vi "PWM Set Frequency.vi"(7 "pPrecision":u16, 8 "error in (no error)":errorcluster, 9 "pPrescaler":u16, 10 "ChannelMask":u8, 11 "DevHandle":i32) -> (0 "error out":errorcluster, 1 "pPrescaler out":u16, 3 "function return":i32, 5 "pPrecision out":u16)   [LabVIEW 2010, in "usb2pwm.lvlib"]
doc: "int WINAPI PWM_SetFrequency(int DevHandle,unsigned char ChannelMask,unsigned short *pPrescaler,unsigned short *pPrecision);"
uses:
  usb2pwm.lvlib
  libs/msvc_x86/USB2XXX.dll
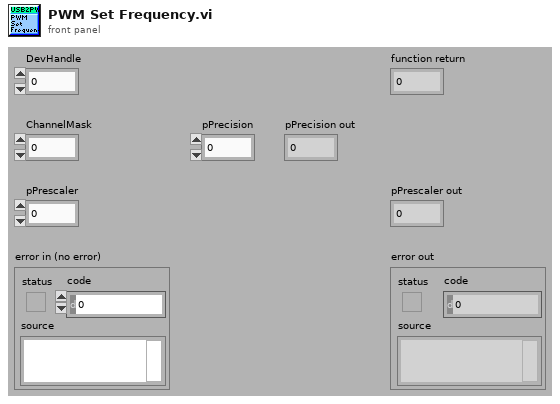
[diagram p1: front panel]
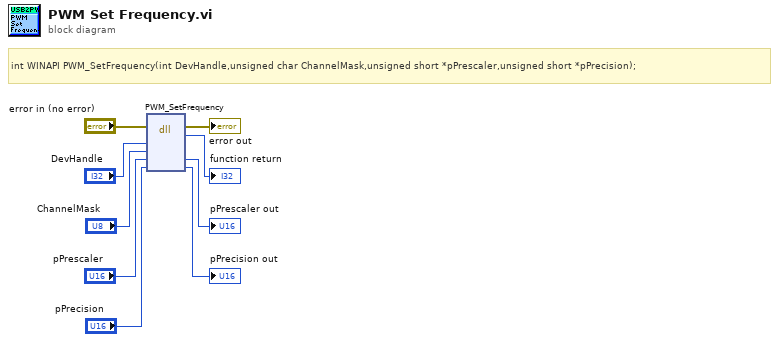
[diagram p0: block diagram]
diagram:
  # "int WINAPI PWM_SetFrequency(int DevHandle,unsigned char ChannelMask,unsigned short *pPrescaler,unsigned short *pPrecision);"
  n1 = dll-call lib="E:/OtherWork/STM32/USB2XXX_Example/sdk/libs/msvc_x86/USB2XXX.*" fn="PWM_SetFrequency"(error in="error in (no error)", "DevHandle"="DevHandle", "ChannelMask"="ChannelMask", "pPrescaler"="pPrescaler", "pPrecision"="pPrecision") -> (error out=→"error out":errorcluster, →"function return":i32, "pPrescaler"=→"pPrescaler out":u16, "pPrecision"=→"pPrecision out":u16)  [unwired: 4 in, 1 out]
